vi "box.vi"(8 "error in (no error)":errorcluster, 11 "Pizza in":refnum<class "Pizza.lvclass">) -> (0 "error out":errorcluster, 2 "boxing message":string, 3 "Pizza out":refnum<class "Pizza.lvclass">)   [LabVIEW 2021, in "Pizza.lvclass"]
uses:
  Pizza.lvclass
panel:
  # "Connector Pane"
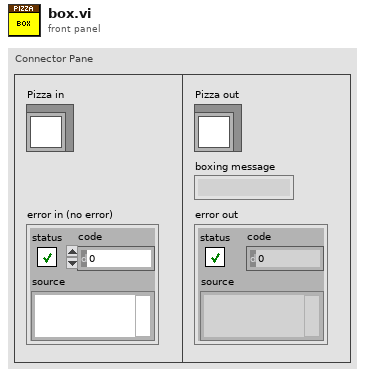
[diagram p1: front panel]
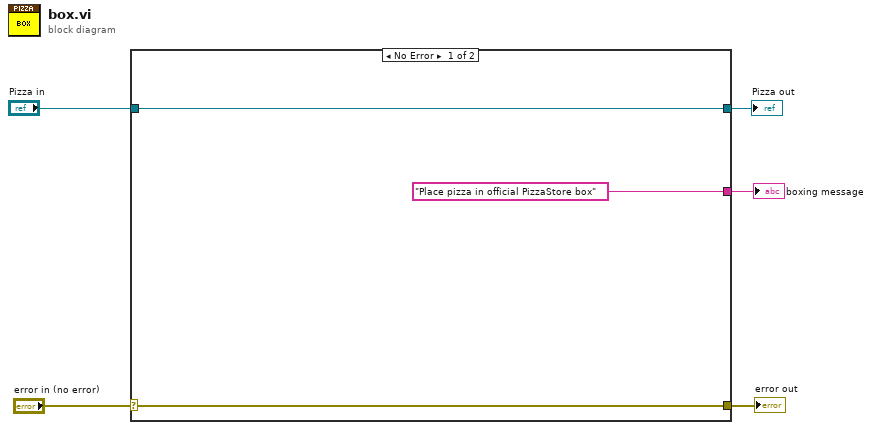
[diagram p0: block diagram]
diagram:
  n1 = case shown="No Error" "error in (no error)" {
    selector: "error in (no error)" -> [w8 w10]
    tunnel: [w8 w10] -> w4
    tunnel: [w7 w9] -> w2
    tunnel: "Pizza in" -> [w7 w9]
    tunnel: ["Place pizza in official PizzaStore box" _] -> w1
    frame No Error {
    }
    frame Error {
    }
  }
  "error out" <- w4
  "Pizza out" <- w2
  "boxing message" <- w1
